vi "7sigment.vi"() -> ()   [LabVIEW 2018]
panel:
  out "NUMBER IN DECIMAL":dbl
  in  "reset":bool
  in  "clock (T/2) ms":u32
  out "Q0":bool=TRUE
  out "Q 1":bool=TRUE
  out "Q 2":bool=TRUE
  out "Q 3":bool=TRUE
  in  "?":u16(ring) items=["up count", "down count"]
  out "E":bool
  out "F":bool
  out "C":bool
  out "B":bool
  out "D":bool
  out "G":bool
  out "A":bool
  # "HEXADECIMAL COUNTER"
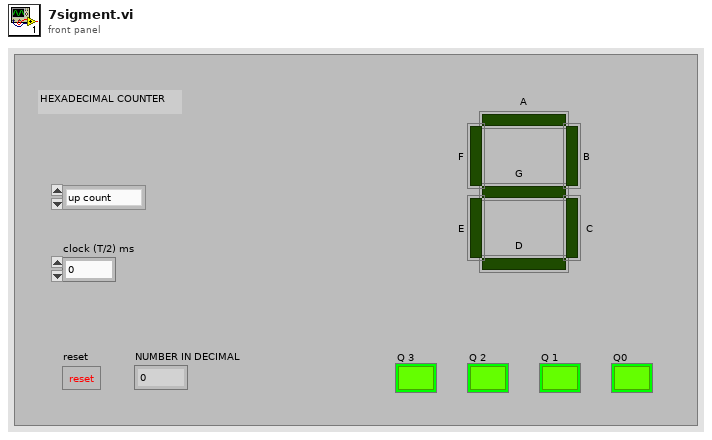
[diagram p1: front panel]
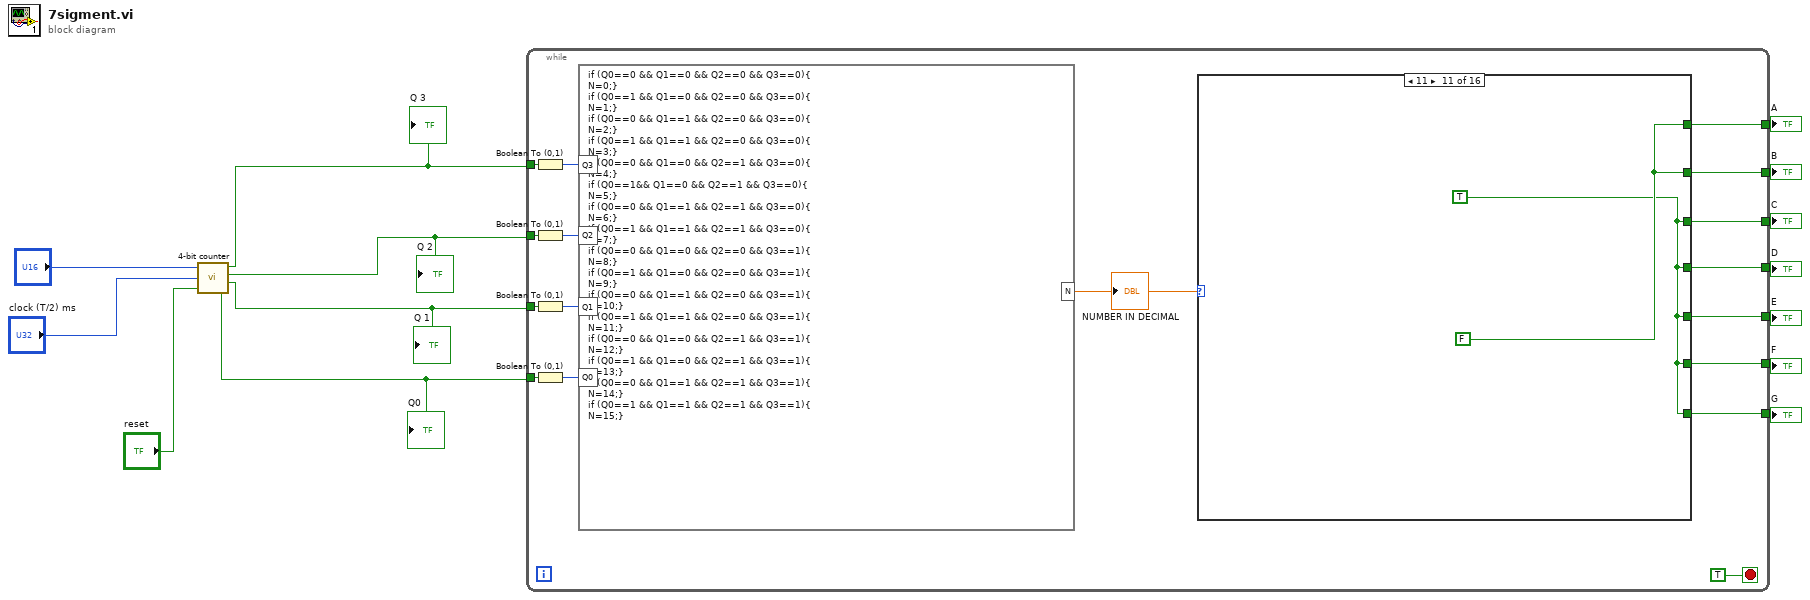
[diagram p0: block diagram]
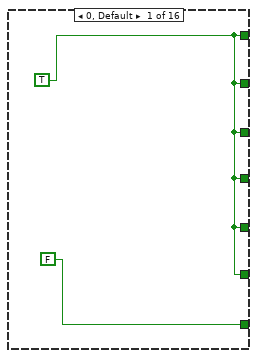
[diagram p2: hidden frame]
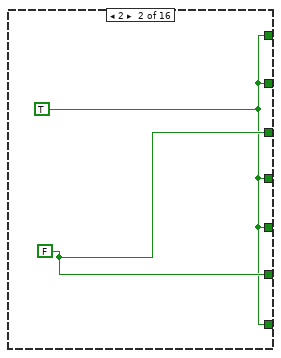
[diagram p3: hidden frame]
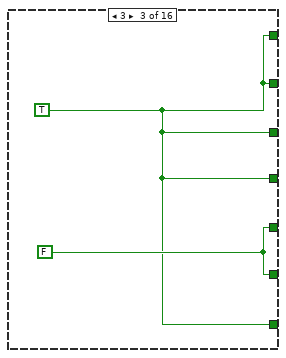
[diagram p4: hidden frame]
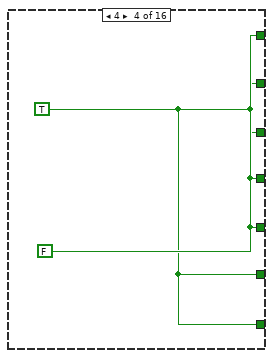
[diagram p5: hidden frame]
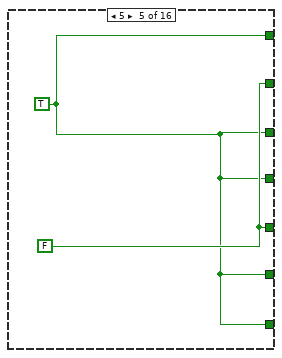
[diagram p6: hidden frame]
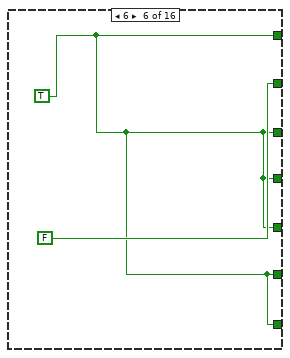
[diagram p7: hidden frame]
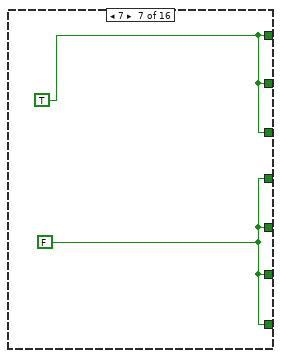
[diagram p8: hidden frame]
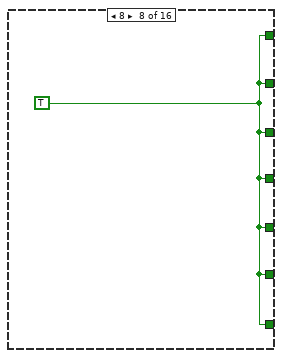
[diagram p9: hidden frame]
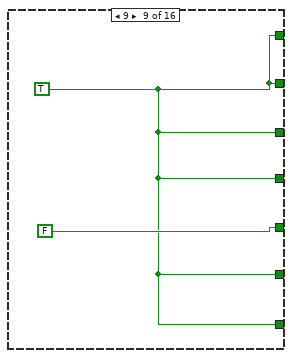
[diagram p10: hidden frame]
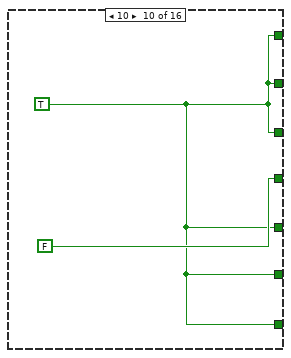
[diagram p11: hidden frame]
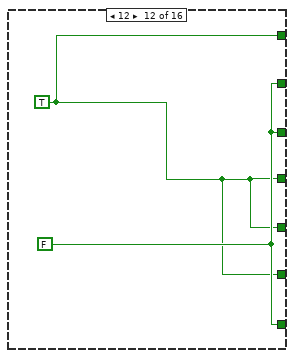
[diagram p12: hidden frame]
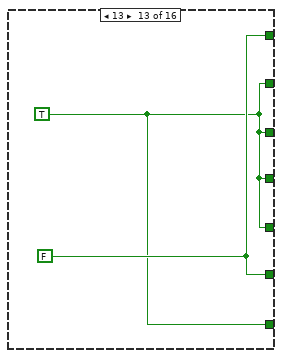
[diagram p13: hidden frame]
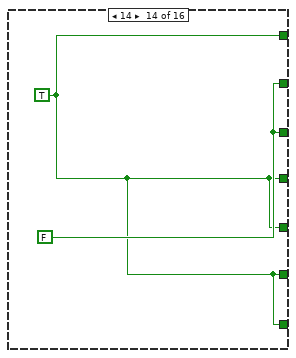
[diagram p14: hidden frame]
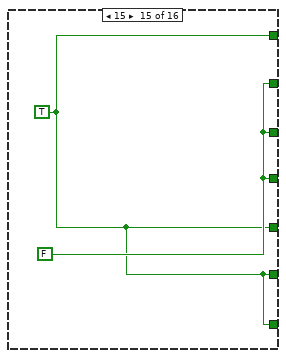
[diagram p15: hidden frame]
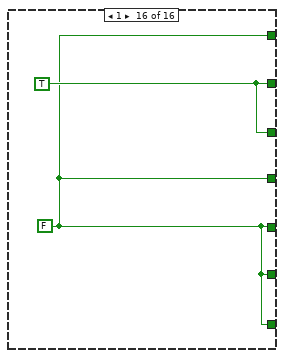
[diagram p16: hidden frame]
diagram:
  n1 = call "4-bit counter.vi"(0:"?", "clock (T/2) ms"="clock (T/2) ms", "reset"="reset") -> ("Q 4"=w5:bool, "Q 3"=w7:bool, "Q 2"=w6:bool, "Q"=w4:bool)
  "Q 3" <- w5
  "Q 2" <- w7
  "Q 1" <- w6
  "Q0" <- w4
  n2 = while {
    tunnel: w5 -> [w27]
    tunnel: w7 -> [w26]
    tunnel: w6 -> [w25]
    tunnel: w4 -> [w24]
    tunnel: [w21] -> w14
    tunnel: [w22] -> w13
    tunnel: [w20] -> w12
    tunnel: [w19] -> w11
    tunnel: [w18] -> w10
    tunnel: [w17] -> w9
    tunnel: [w16] -> w8
    stop <- TRUE stop-if-true
    n3 = Boolean To (0,1)(Boolean=w27) -> (0, 1=w31:i16)
    n4 = Boolean To (0,1)(Boolean=w26) -> (0, 1=w30:i16)
    n5 = Boolean To (0,1)(Boolean=w25) -> (0, 1=w29:i16)
    n6 = Boolean To (0,1)(Boolean=w24) -> (0, 1=w28:i16)
    n7 = formula code="if (Q0==0 && Q1==0 && Q2==0 && Q3==0){\nN=0;}\nif (Q0==1 && Q1==0 && Q2==0 && Q3==0){\nN=1;}\nif (Q0==0 && Q1==1 && Q2==0 && Q3==0){\nN=2;}\nif (Q0==1 && Q1==1 && Q2==0 && Q3==0){\nN=3;}\nif (Q0==0 && Q1==0 && Q2==1 && Q3==0){\nN=4;}\nif (Q0==1&& Q1==0 && Q2==1 && Q3==0){\nN=5;}\nif (Q0==0 && Q1==1 && Q2==1 && Q3==0){\nN=6;}\nif (Q0==1 && Q1==1 && Q2==1 && Q3==0){\nN=7;}\nif (Q0==0 && Q1==0 && Q2==0 && Q3==1){\nN=8;}\nif (Q0==1 && Q1==0 && Q2==0 && Q3==1){\nN=9;}\nif (Q0==0 && Q1==1 && Q2==0 && Q3==1){\nN=10;}\nif (Q0==1 && Q1==1 && Q2==0 && Q3==1){\nN=11;}\nif (Q0==0 && Q1==0 && Q2==1 && Q3==1){\nN=12;}\nif (Q0==1 && Q1==0 && Q2==1 && Q3==1){\nN=13;}\nif (Q0==0 && Q1==1 && Q2==1 && Q3==1){\nN=14;}\nif (Q0==1 && Q1==1 && Q2==1 && Q3==1){\nN=15;}"("Q3"=w31, "Q2"=w30, "Q1"=w29, "Q0"=w28) -> ("N"=w15:dbl)
    "NUMBER IN DECIMAL" <- w15
    n8 = case shown="11" w15 {
      tunnel: [w33 w34 w36 w39 w40 w42 w45 w46 w47 w49 w52 w53 w56 w57 w59 w61] -> w22
      tunnel: [w33 w34 w36 w38 w41 FALSE w45 w46 w47 w49 w52 w54 w55 w58 w60 w62] -> w21
      tunnel: [w33 w35 w36 w38 w40 w42 w45 w46 w47 w49 w51 w54 w55 w58 w60 w62] -> w20
      tunnel: [w33 w34 w36 w39 w40 w42 w44 w46 w47 FALSE w51 w53 w55 w57 w60 w61] -> w19
      tunnel: [w33 w34 w37 w39 w41 w42 w44 w46 FALSE w49 w51 w53 w55 w57 w59 w61] -> w18
      tunnel: [w33 w35 w37 w38 w40 w42 w44 w46 w47 w49 w51 w53 w56 w57 w59 w61] -> w17
      tunnel: [FALSE w34 w36 w38 w40 w42 w44 w46 w47 w49 w51 w54 w55 w57 w59 w61] -> w16
      frame 0, Default {
        w33 = TRUE
      }
      frame 2 {
        w35 = FALSE
        w34 = TRUE
      }
      frame 3 {
        w37 = FALSE
        w36 = TRUE
      }
      frame 4 {
        w39 = FALSE
        w38 = TRUE
      }
      frame 5 {
        w41 = FALSE
        w40 = TRUE
      }
      frame 6 {
        w42 = TRUE
      }
      frame 7 {
        w44 = FALSE
        w45 = TRUE
      }
      frame 8 {
        w46 = TRUE
      }
      frame 9 {
        w47 = TRUE
      }
      frame 10 {
        w49 = TRUE
      }
      frame 11 {
        w52 = FALSE
        w51 = TRUE
      }
      frame 12 {
        w54 = FALSE
        w53 = TRUE
      }
      frame 13 {
        w56 = FALSE
        w55 = TRUE
      }
      frame 14 {
        w58 = FALSE
        w57 = TRUE
      }
      frame 15 {
        w60 = FALSE
        w59 = TRUE
      }
      frame 1 {
        w61 = FALSE
        w62 = TRUE
      }
    }
  }
  "A" <- w13
  "G" <- w8
  "D" <- w11
  "B" <- w14
  "C" <- w12
  "F" <- w9
  "E" <- w10
